vi "Create Wrapper for Measurement Plugin.vi"(11 "error in (no error)":errorcluster) -> (15 "error out":errorcluster)   [LabVIEW 2021, in "Converter.lvlib"]
uses:
  Converter.lvlib
  <vilib>/Utility/miscctls.llb/LVPointTypeDef.ctl
  <vilib>/Utility/traverseref.llb/TRef TravTarget.ctl
  <vilib>/Utility/traverseref.llb/VI Scripting - Traverse.lvlib
  Converter Reusables/Converter Reusables.lvlib
  Path Functions/Path Functions.lvlib
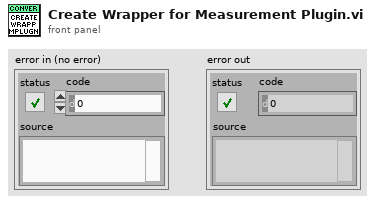
[diagram p1: front panel]
types:
  T1 = typedef "TRef TravTarget.ctl" = enum16{"FP", "BD", "Other"}
  T2 = typedef "LVPointTypeDef.ctl" = cluster{"Horizontal":i16, "Vertical":i16}
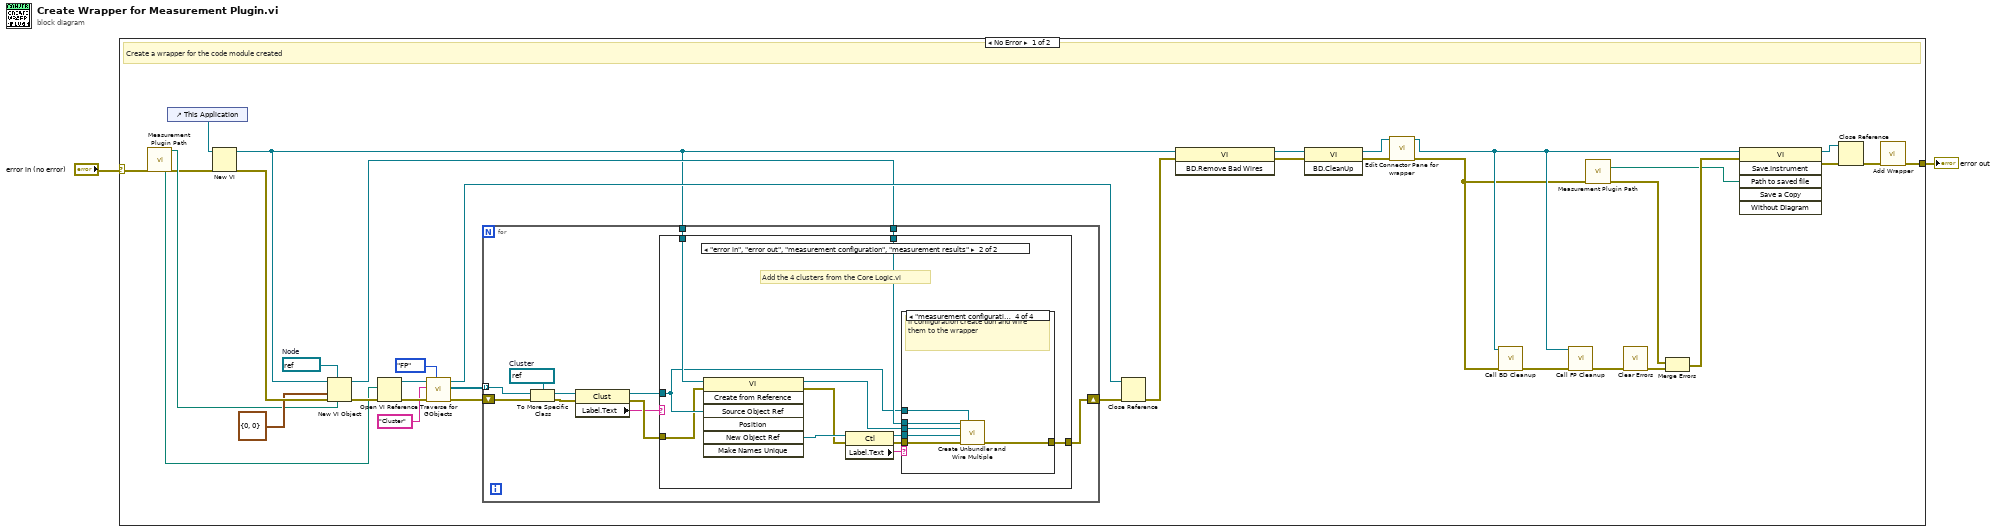
[diagram p0: block diagram]
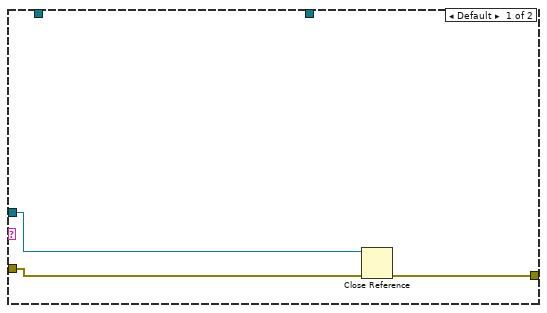
[diagram p2: hidden frame]
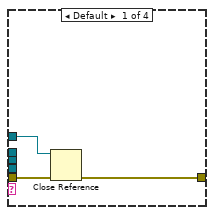
[diagram p3: hidden frame]
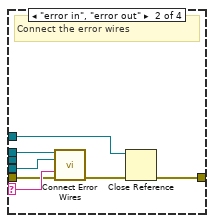
[diagram p4: hidden frame]
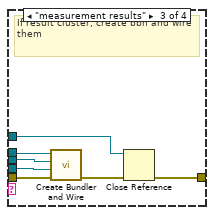
[diagram p5: hidden frame]
diagram:
  n1 = case shown="No Error" "error in (no error)" {
    selector: "error in (no error)" -> [w9 w87]
    tunnel: [w3 w87] -> w2
    frame No Error {
      w38 = refnum<vi> refnum  # Node
      # "Create a wrapper for the code module created"
      n2 = call "Measurement Plugin Path.vi"("error in (no error)"=w9) -> ("New Code Module"=w11:path, "Logic VI Path"=w10:path, "error out"=w8:errorcluster)  [unwired: 2 in, 10 out]
      n3 = control-ref of="This Application"() -> (w23:refnum<vi>)
      n4 = New VI(8:w8, 11:w23) -> (0:w37:errorcluster, 3:w22:refnum<vi>)  [unwired: 5 in]
      n5 = New VI Object(vi object class=w38, owner refnum=w22, position/next to=T2 {"Horizontal"=0, "Vertical"=0} ("location"), 6:w11, 8:w37) -> (object refnum=w24:refnum<vi>, 0:w33:errorcluster)  [unwired: 3 in]
      n6 = Open VI Reference(vi path=w10, error in (no error)=w33) -> (vi reference=w29:refnum<vi>, error out=w32:errorcluster)  [unwired: 4 in]
      n7 = call <vilib>:"Traverse for GObjects.vi"("Traverse Target"=TRef_TravTarget."FP", "error in (no error)"=w32, "Class Name"="Cluster", "VI Refnum"=w29) -> ("error out"=w30:errorcluster, "References"=w27:refnum<vi>[], "dup VI Refnum"=w26:refnum<vi>)  [unwired: 4 in, 1 out]
      n8 = for {
        shift-right: [w45] -> w28
        shift-left: w30 -> [w48]
        tunnel: w27 -> [w44] mode=indexing
        tunnel: w22 -> [w47]
        tunnel: w24 -> [w46]
        w49 = refnum<vi> refnum  # Cluster
        n9 = To More Specific Class(target class=w49, reference=w44, error in=w48) -> (specific class reference=w41:refnum<vi>, error out=w43:errorcluster)
        n10 = property class="Clust"(reference=w41, error in=w43) -> (reference out=w40:refnum<vi>, error out=w42:errorcluster, "Label.Text"=w39:string)
        n11 = case shown="\"error in\", \"error out\", \"measurement configuration\", \"measurement results\"" w39 {
          tunnel: w47 -> [_ w63]
          tunnel: w46 -> [_ w57]
          tunnel: [w51 w56] -> w45
          tunnel: w40 -> [w50 w54]
          tunnel: w42 -> [w52 w53]
          frame Default {
            n12 = Close Reference(reference=w50, error in (no error)=w52) -> (error out=w51:errorcluster)
          }
          frame "error in", "error out", "measurement configuration", "measurement results" {
            # "Add the 4 clusters from the Core Logic.vi"
            n13 = invoke class="VI" method="Create from Reference"(reference=w63, error in=w53, "Source Object Ref"=w54) -> (reference out=w58:refnum<vi>, error out=w61:errorcluster, "New Object Ref"=w62:refnum<vi>)  [unwired: 4 in, 4 out]
            n14 = property class="Ctl"(reference=w62, error in=w61) -> (reference out=w55:refnum<vi>, error out=w60:errorcluster, "Label.Text"=w59:string)
            n15 = case shown="\"measurement configuration\"" w59 {
              selector: w59 -> [_ w72 _ _]
              tunnel: w60 -> [w66 w69 w80 w85]
              tunnel: w58 -> [_ _ w79 w82]
              tunnel: w57 -> [_ w73 w78 w83]
              tunnel: [w64 w68 w75 w86] -> w56
              tunnel: w54 -> [w65 w67 w74 w84]
              tunnel: w55 -> [_ w70 w76 w81]
              frame Default {
                n16 = Close Reference(reference=w65, error in (no error)=w66) -> (error out=w64:errorcluster)
              }
              frame "error in", "error out" {
                # "Connect the error wires"
                n17 = call "Connect Error Wires.vi"("Node in"=w73, "New Object Ref"=w70, "String"=w72, "error in (no error)"=w69) -> ("error out"=w71:errorcluster)  [unwired: 11 in]
                n18 = Close Reference(reference=w67, error in (no error)=w71) -> (error out=w68:errorcluster)
              }
              frame "measurement results" {
                # "If result cluster, create bbn and wire them"
                n19 = call "Create Bundler and Wire.vi"("error in (no error)"=w80, "New Object Ref"=w76, "vi refnum"=w79, "Node in"=w78) -> ("error out"=w77:errorcluster)  [unwired: 7 in]
                n20 = Close Reference(reference=w74, error in (no error)=w77) -> (error out=w75:errorcluster)
              }
              frame "measurement configuration" {
                # "If configuration create ubn and wire them to the wrapper"
                n21 = call "Create Unbundler and Wire Multiple.vi"("Node in"=w83, "Clust Refnum"=w84, "vi refnum"=w82, "New Object Ref"=w81, "error in (no error)"=w85) -> ("error out"=w86:errorcluster)  [unwired: 10 in]
              }
            }
          }
        }
      }
      n22 = Close Reference(reference=w26, error in (no error)=w28) -> (error out=w19:errorcluster)
      n23 = invoke class="VI" method="BD.Remove Bad Wires"(reference=w22, error in=w19) -> (reference out=w21:refnum<vi>, error out=w20:errorcluster)  [unwired: 1 in, 1 out]
      n24 = invoke class="VI" method="BD.CleanUp"(reference=w21, error in=w20) -> (reference out=w14:refnum<vi>, error out=w12:errorcluster)  [unwired: 1 in, 1 out]
      n25 = call "Edit Connector Pane for wrapper.vi"("vi reference"=w14, "error in (no error)"=w12) -> ("vi reference out"=w13:refnum<vi>, "error out"=w6:errorcluster)  [unwired: 12 in]
      n26 = call "Call BD Cleanup.vi"("VI"=w13, "error in (no error)"=w6) -> ("error out"=w18:errorcluster)  [unwired: 13 in]
      n27 = call "Call FP Cleanup.vi"("VI"=w13, "error in (no error)"=w18) -> ("error out"=w17:errorcluster)  [unwired: 13 in]
      n28 = call "Measurement Plugin Path.vi"("error in (no error)"=w6) -> ("Wrapper Path"=w7:path, "error out"=w5:errorcluster)  [unwired: 2 in, 11 out]
      n29 = call <vilib>:"Clear Errors.vi"("error in (no error)"=w17) -> ("error out"=w16:errorcluster)  [unwired: 5 in, 1 out]
      n30 = Merge Errors(w5, w16) -> (w15:errorcluster)
      n31 = invoke class="VI" method="Save.Instrument"(reference=w13, error in=w15, "Path to saved file"=w7) -> (reference out=w34:refnum<vi>, error out=w35:errorcluster)  [unwired: 3 in, 4 out]
      n32 = Close Reference(reference=w34, error in (no error)=w35) -> (error out=w4:errorcluster)
      n33 = call "Add Wrapper.vi"("error in (no error)"=w4) -> ("error out"=w3:errorcluster)  [unwired: 14 in]
    }
    frame Error {
    }
  }
  "error out" <- w2
